vi "Autonomous Independent.vi"   [LabVIEW 2019]
doc: "This VI is called when autonomous begins, and will automatically be terminated when autonomous ends. You can carry out timed or sensor driven robot movement independently without needing to return to the caller."
uses:
  <vilib>/Rock Robotics/WPI/SafetyOutput/WPI_SafetyOutputConfigMenu.ctl
  <vilib>/Rock Robotics/WPI/Solenoid/WPI_SolenoidValue.ctl
  <vilib>/Rock Robotics/WPI/Utilities/WPI_GetSetVariantRefNum.vi
  <vilib>/Rock Robotics/Network Tables/NT Read String.vi
  <vilib>/Rock Robotics/Network Tables/NT Write Numeric Array.vi
  <vilib>/Rock Robotics/WPI/Solenoid/WPI_SolenoidSetEnum.vi
  <vilib>/Rock Robotics/WPI/RobotDrive/WPI_RobotDriveArcadeDrive_Standard(NoSaturation).vi
panel:
  # "Be sure to right-click and choose Data Operations>>Make Current Value default if you want to save the array values with the VI"
types:
  T1 = typedef "WPI_JoystickDevRef.ctl" = cluster{"Device":T2}
  T2 = typedef "WPI_JoystickDeviceEnum.ctl" = enum16{"USB 0", "USB 1", "USB 2", "USB 3", "USB 4", "USB 5"}
  T3 = typedef "WPI_SafetyOutputConfigMenu.ctl" = enum16{"Enable", "Disable"}
  T4 = typedef "WPI_SolenoidValue.ctl" = enum16{"Off", "On", "Forward", "Reverse"}
  T5 = typedef "WPI_RobotDriveDevRef.ctl" = cluster{"DevStatus":errorcluster, "Motors[]":T6[], "Square Inputs":bool, "Max Output":dbl}
  T6 = typedef "WPI_MotorControlDeviceRef.ctl" = cluster{"DeviceStatus":errorcluster, "Type":T7, "PWM":cluster{"PWM Channel":T8, "DeadBand":T9}, "CAN":cluster{"Device Number":u8, "SetOutput VI Ref":variant, "GetOutput VI Ref":variant, "Enable VI Ref":variant, "Disable VI Ref":variant, "Data":variant}, "Invert":bool, "DIO PWM":cluster{"PWM \"Enable\" Channel":T8, "DIOChannel":T10, "PWM Rate":dbl}}
  T7 = typedef "WPI_MotorControlType.ctl" = enum16{"PWM", "CAN", "DIO PWM"}
  T8 = typedef "FPGA_DIOPWMChannel.ctl" = enum8{"PWM 0", "PWM 1", "PWM 2", "PWM 3", "PWM 4", "PWM 5", "PWM 6", "PWM 7", "PWM 8", "PWM 9", "PWM MXP 0", "PWM MXP 1", "PWM MXP 2", "PWM MXP 3", "PWM MXP 4", "PWM MXP 5", "PWM MXP 6", "PWM MXP 7", "PWM MXP 8", "PWM MXP 9", "Invalid"}
  T9 = typedef "WPI_PWMDeadband.ctl" = cluster{"Name":string, "maxPositivePwm":i32, "minPositivePwm":i32, "centerPwm":i32, "maxNegativePwm":i32, "minNegativePwm":i32, "angularRange":u16}
  T10 = typedef "FPGA_DIOChannel.ctl" = enum8{"DIO 0", "DIO 1", "DIO 2", "DIO 3", "DIO 4", "DIO 5", "DIO 6", "DIO 7", "DIO 8", "DIO 9", "DIO MXP 0", "DIO MXP 1", "DIO MXP 2", "DIO MXP 3", "DIO MXP 4", "DIO MXP 5", "DIO MXP 6", "DIO MXP 7", "DIO MXP 8", "DIO MXP 9", "DIO MXP 10", "DIO MXP 11", "DIO MXP 12", "DIO MXP 13", "DIO MXP 14", "DIO MXP 15", "SPI Port CS1", "SPI Port CS2", "SPI Port CS3", "SPI Port MISO", "SPI Port MOSI", "Invalid"}
  T11 = typedef "WPI_SolenoidDevRef.ctl" = cluster{"DevStatus":errorcluster, "Pneumatics Control Module":u8, "Forward Solenoid Channel":T12, "Reverse Solenoid Channel":T12}
  T12 = typedef "WPI_SolenoidChannel.ctl" = enum8{"Solenoid 0", "Solenoid 1", "Solenoid 2", "Solenoid 3", "Solenoid 4", "Solenoid 5", "Solenoid 6", "Solenoid 7", "Invalid"}
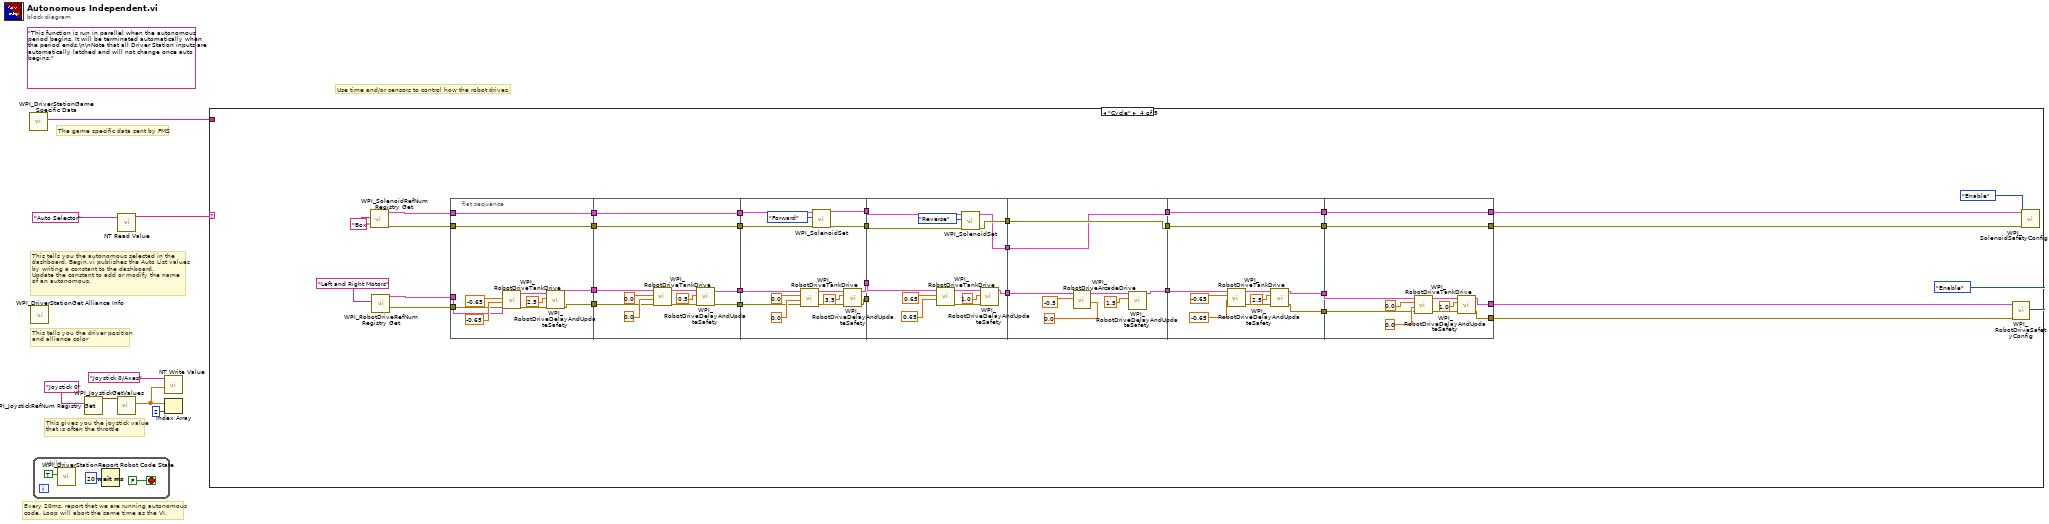
[diagram p0: block diagram]
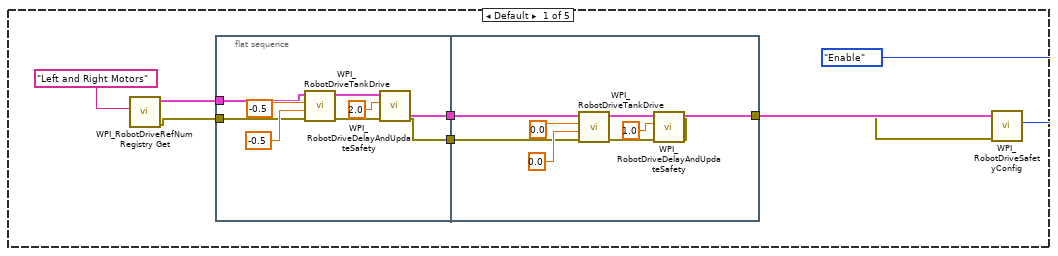
[diagram p2: hidden frame]
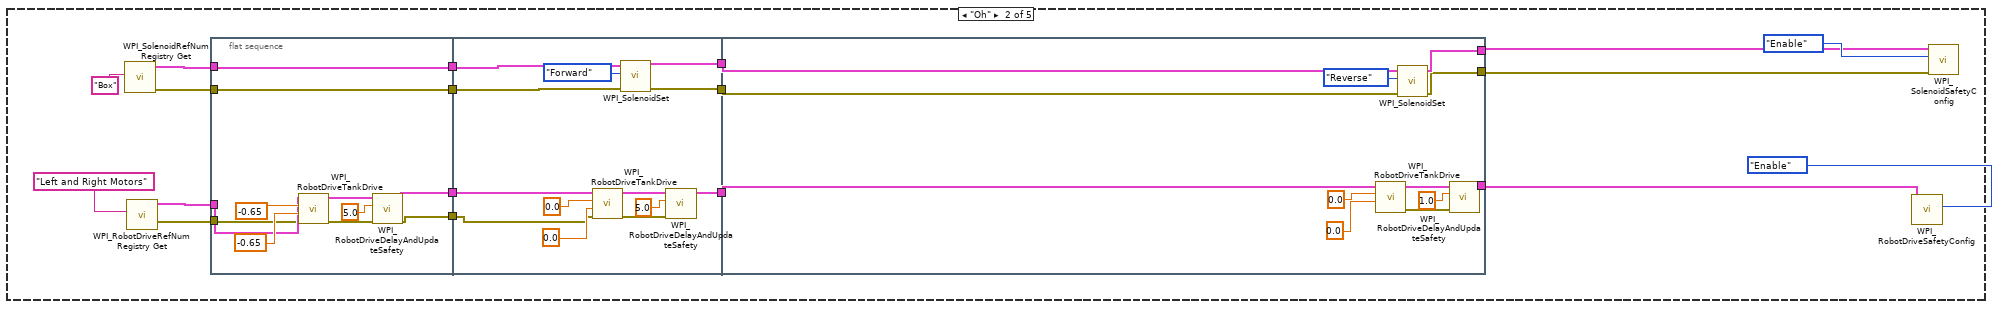
[diagram p3: hidden frame]
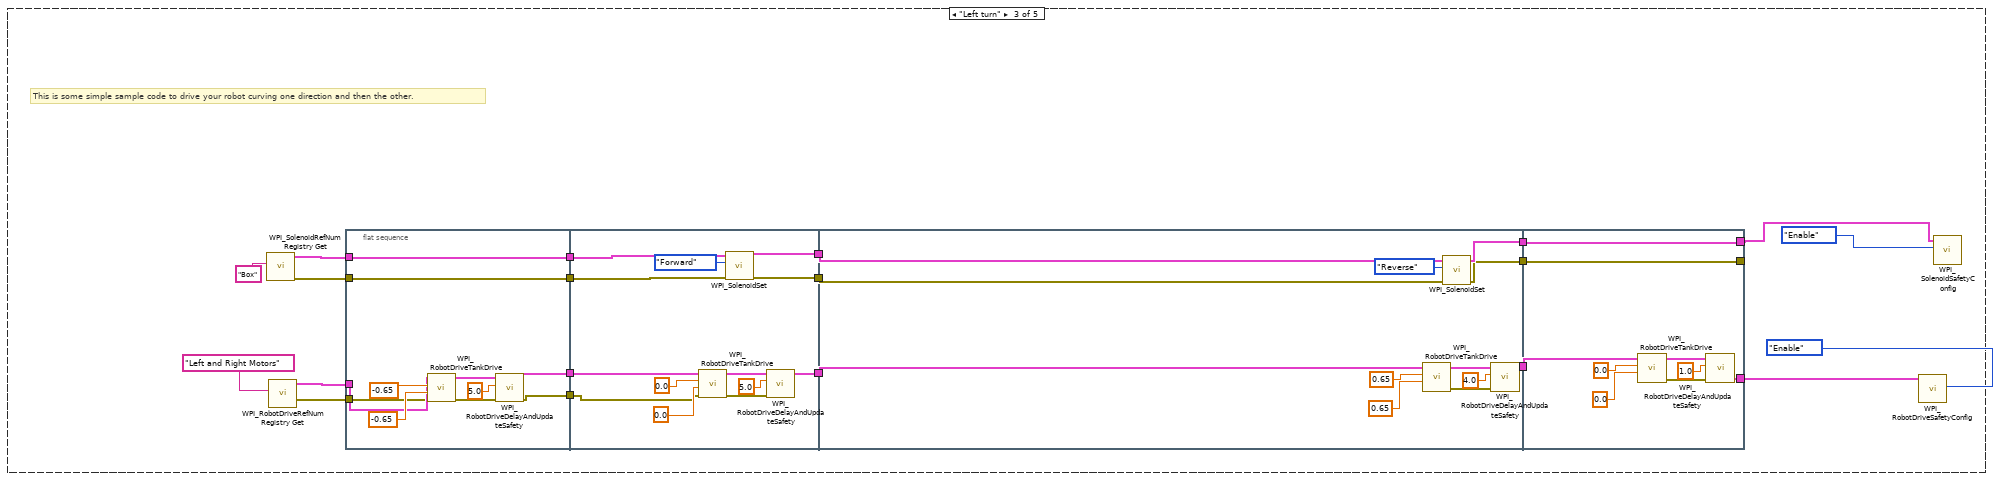
[diagram p4: hidden frame]
diagram:
  (unwired) "This function is run in parallel when the autonomous period begins. It will be terminated automatically when the period ends.\n\nNote that all Driver Station inputs are automatically latched and will not change once auto begins."
  # "The game specific data sent by FMS"
  # "This tells you the autonomous selected in the \ndashboard. Begin.vi publishes the Auto List values\nby writing a constant to the dashboard.\nUpdate the constant to add or modify the name\nof an autonomous."
  # "Every 20ms, report that we are running autonomous\ncode. Loop will abort the same time as the VI."
  # "This gives you the joystick value\nthat is often the throttle"
  # "Use time and/or sensors to control how the robot drives."
  # "This tells you the driver position\nand alliance color"
  n1 = call <vilib>:"WPI_DriverStationGame Specific Data.vi"() -> ("Game Specific Data"=w1:string)  [unwired: 11 in]
  n2 = call <vilib>:"WPI_DriverStationGet Alliance Info.vi"() -> ()  [unwired: 12 out]
  n3 = while {
    stop <- FALSE stop-if-true
    n4 = call <vilib>:"WPI_DriverStationReport Robot Code State.vi"("Autonomous"=TRUE) -> ()  [unwired: 10 in, 1 out]
    n5 = Wait (ms)(milliseconds to wait=u32 20) -> ()  [unwired: 1 out]
  }
  n6 = call <vilib>:"WPI_JoystickRefNum Registry Get.vi"("refnum name"="Joystick 0") -> ("JoystickDevRef"=w7:T1)  [unwired: 1 in, 9 out]
  n7 = call <vilib>:"WPI_JoystickGetValues.vi"("JoystickDevRef"=w7) -> ("Axes"=w3:dbl[])  [unwired: 6 in, 4 out]
  n8 = call-poly <vilib>:"NT Read Value.vi"("Name"="Auto Selector") -> ("String"=w4:string)  [unwired: 9 in, 1 out]
  n9 = call-poly <vilib>:"NT Write Value.vi"("Numeric Array"=w3, "Name"="Joystick 0/Axes") -> ()  [unwired: 9 in, 1 out]
  n10 = Index Array(array=w3, index=2) -> ()  [unwired: 1 out]
  n11 = case shown="\"Cycle\"" w4 {
    tunnel: w1 -> [_ _ _ _ _]
    frame Default {
      n12 = call <vilib>:"WPI_RobotDriveRefNum Registry Get.vi"("refnum name"="Left and Right Motors") -> ("error out"=w12:errorcluster, "RobotDriveDevRef"=w18:T5)  [unwired: 1 in, 8 out]
      n13 = flat-sequence {
        tunnel: w18 -> [w23]
        tunnel: [w22] -> w17
        tunnel: [w21] -> w13
        tunnel: w12 -> [w20]
        tunnel: w17 -> [w32]
        tunnel: [w31] -> w15
        tunnel: [w30] -> w14
        tunnel: w13 -> [w29]
        frame #0 {
          n14 = call <vilib>:"WPI_RobotDriveTankDrive.vi"("error in (no error)"=w20, "Right axis value"=-0.5 ("X axis value"), "Left axis value"=-0.5 ("X axis value"), "RobotDriveDevRef"=w23) -> ("error out"=w24:errorcluster, "RobotDriveDevRef"=w27:T5)  [unwired: 5 in, 1 out]
          n15 = call <vilib>:"WPI_RobotDriveDelayAndUpdateSafety.vi"("error in (no error)"=w24, "Delay (s)"=2.0, "RobotDriveDevRef"=w27) -> ("error out"=w21:errorcluster, "RobotDriveDevRef 2"=w22:T5)  [unwired: 7 in]
        }
        frame #1 {
          n16 = call <vilib>:"WPI_RobotDriveTankDrive.vi"("error in (no error)"=w29, "Right axis value"=0.0 ("X axis value"), "Left axis value"=0.0 ("X axis value"), "RobotDriveDevRef"=w32) -> ("error out"=w33:errorcluster, "RobotDriveDevRef"=w36:T5)  [unwired: 5 in, 1 out]
          n17 = call <vilib>:"WPI_RobotDriveDelayAndUpdateSafety.vi"("error in (no error)"=w33, "Delay (s)"=1.0, "RobotDriveDevRef"=w36) -> ("error out"=w30:errorcluster, "RobotDriveDevRef 2"=w31:T5)  [unwired: 7 in]
        }
      }
      n18 = call <vilib>:"WPI_RobotDriveSafetyConfig.vi"("error in (no error)"=w14, "mode"=WPI_SafetyOutputConfigMenu."Enable", "RobotDriveDevRef"=w15) -> ()  [unwired: 7 in, 2 out]
    }
    frame "Oh" {
      n19 = call <vilib>:"WPI_SolenoidRefNum Registry Get.vi"("refnum name"="Box") -> ("error out"=w43:errorcluster, "SolenoidDevRef"=w52:T11)  [unwired: 9 in]
      n20 = call <vilib>:"WPI_RobotDriveRefNum Registry Get.vi"("refnum name"="Left and Right Motors") -> ("error out"=w45:errorcluster, "RobotDriveDevRef"=w53:T5)  [unwired: 1 in, 8 out]
      n21 = flat-sequence {
        tunnel: w53 -> [w61]
        tunnel: w52 -> [w60]
        tunnel: [w60] -> w51
        tunnel: [w59] -> w50
        tunnel: [w58] -> w46
        tunnel: w45 -> [w57]
        tunnel: [w56] -> w44
        tunnel: w43 -> [w56]
        tunnel: [w78] -> w49
        tunnel: [w76] -> w42
        tunnel: [w69] -> w40
        tunnel: w44 -> [w77]
        tunnel: w46 -> [w67]
        tunnel: w50 -> [w70]
        tunnel: w51 -> [w79]
        tunnel: [w85] -> w41
        tunnel: [w84] -> w39
        tunnel: [w83] -> w38
        tunnel: w49 -> [w82]
        tunnel: w42 -> [w80]
        tunnel: w40 -> [w81]
        frame #0 {
          n22 = call <vilib>:"WPI_RobotDriveTankDrive.vi"("error in (no error)"=w57, "Right axis value"=-0.65 ("X axis value"), "Left axis value"=-0.65 ("X axis value"), "RobotDriveDevRef"=w61) -> ("error out"=w62:errorcluster, "RobotDriveDevRef"=w65:T5)  [unwired: 5 in, 1 out]
          n23 = call <vilib>:"WPI_RobotDriveDelayAndUpdateSafety.vi"("error in (no error)"=w62, "Delay (s)"=5.0, "RobotDriveDevRef"=w65) -> ("error out"=w58:errorcluster, "RobotDriveDevRef 2"=w59:T5)  [unwired: 7 in]
        }
        frame #1 {
          n24 = call <vilib>:"WPI_RobotDriveTankDrive.vi"("error in (no error)"=w67, "Right axis value"=0.0 ("X axis value"), "Left axis value"=0.0 ("X axis value"), "RobotDriveDevRef"=w70) -> ("error out"=w75:errorcluster, "RobotDriveDevRef"=w74:T5)  [unwired: 5 in, 1 out]
          n25 = call-poly <vilib>:"WPI_SolenoidSet.vi"("error in (no error)"=w77, "Value"=WPI_SolenoidValue."Forward", "SolenoidDevRef"=w79) -> ("error out"=w76:errorcluster, "SolenoidDevRef"=w78:T11)  [unwired: 7 in]
          n26 = call <vilib>:"WPI_RobotDriveDelayAndUpdateSafety.vi"("error in (no error)"=w75, "Delay (s)"=5.0, "RobotDriveDevRef"=w74) -> ("RobotDriveDevRef 2"=w69:T5)  [unwired: 7 in, 1 out]
        }
        frame #2 {
          n27 = call <vilib>:"WPI_RobotDriveTankDrive.vi"("Right axis value"=0.0 ("X axis value"), "Left axis value"=0.0 ("X axis value"), "RobotDriveDevRef"=w81) -> ("error out"=w90:errorcluster, "RobotDriveDevRef"=w89:T5)  [unwired: 6 in, 1 out]
          n28 = call-poly <vilib>:"WPI_SolenoidSet.vi"("error in (no error)"=w80, "Value"=WPI_SolenoidValue."Reverse", "SolenoidDevRef"=w82) -> ("error out"=w83:errorcluster, "SolenoidDevRef"=w85:T11)  [unwired: 7 in]
          n29 = call <vilib>:"WPI_RobotDriveDelayAndUpdateSafety.vi"("error in (no error)"=w90, "Delay (s)"=1.0, "RobotDriveDevRef"=w89) -> ("RobotDriveDevRef 2"=w84:T5)  [unwired: 7 in, 1 out]
        }
      }
      n30 = call <vilib>:"WPI_RobotDriveSafetyConfig.vi"("mode"=WPI_SafetyOutputConfigMenu."Enable", "RobotDriveDevRef"=w39) -> ()  [unwired: 8 in, 2 out]
      n31 = call <vilib>:"WPI_SolenoidSafetyConfig.vi"("error in (no error)"=w38, "mode"=WPI_SafetyOutputConfigMenu."Enable", "SolenoidDevRef"=w41) -> ()  [unwired: 7 in, 2 out]
    }
    frame "Left turn" {
      # "This is some simple sample code to drive your robot curving one direction and then the other."
      n32 = call <vilib>:"WPI_SolenoidRefNum Registry Get.vi"("refnum name"="Box") -> ("error out"=w97:errorcluster, "SolenoidDevRef"=w101:T11)  [unwired: 9 in]
      n33 = call <vilib>:"WPI_RobotDriveRefNum Registry Get.vi"("refnum name"="Left and Right Motors") -> ("error out"=w98:errorcluster, "RobotDriveDevRef"=w102:T5)  [unwired: 1 in, 8 out]
      n34 = flat-sequence {
        tunnel: w102 -> [w117]
        tunnel: w101 -> [w116]
        tunnel: [w116] -> w108
        tunnel: [w115] -> w109
        tunnel: [w114] -> w110
        tunnel: w98 -> [w113]
        tunnel: [w112] -> w111
        tunnel: w97 -> [w112]
        tunnel: [w134] -> w107
        tunnel: [w132] -> w106
        tunnel: [w125] -> w105
        tunnel: w111 -> [w133]
        tunnel: w110 -> [w123]
        tunnel: w109 -> [w126]
        tunnel: w108 -> [w135]
        tunnel: w107 -> [w138]
        tunnel: w106 -> [w136]
        tunnel: w105 -> [w137]
        tunnel: [w141] -> w96
        tunnel: [w140] -> w95
        tunnel: [w139] -> w94
        tunnel: [w155] -> _
        tunnel: [w156] -> w93
        tunnel: w96 -> [w156]
        tunnel: w95 -> [w149]
        tunnel: w94 -> [w155]
        tunnel: [w148] -> w92
        frame #0 {
          n35 = call <vilib>:"WPI_RobotDriveTankDrive.vi"("error in (no error)"=w113, "Right axis value"=-0.65 ("X axis value"), "Left axis value"=-0.65 ("X axis value"), "RobotDriveDevRef"=w117) -> ("error out"=w118:errorcluster, "RobotDriveDevRef"=w121:T5)  [unwired: 5 in, 1 out]
          n36 = call <vilib>:"WPI_RobotDriveDelayAndUpdateSafety.vi"("error in (no error)"=w118, "Delay (s)"=5.0, "RobotDriveDevRef"=w121) -> ("error out"=w114:errorcluster, "RobotDriveDevRef 2"=w115:T5)  [unwired: 7 in]
        }
        frame #1 {
          n37 = call <vilib>:"WPI_RobotDriveTankDrive.vi"("error in (no error)"=w123, "Right axis value"=0.0 ("X axis value"), "Left axis value"=0.0 ("X axis value"), "RobotDriveDevRef"=w126) -> ("error out"=w131:errorcluster, "RobotDriveDevRef"=w130:T5)  [unwired: 5 in, 1 out]
          n38 = call-poly <vilib>:"WPI_SolenoidSet.vi"("error in (no error)"=w133, "Value"=WPI_SolenoidValue."Forward", "SolenoidDevRef"=w135) -> ("error out"=w132:errorcluster, "SolenoidDevRef"=w134:T11)  [unwired: 7 in]
          n39 = call <vilib>:"WPI_RobotDriveDelayAndUpdateSafety.vi"("error in (no error)"=w131, "Delay (s)"=5.0, "RobotDriveDevRef"=w130) -> ("RobotDriveDevRef 2"=w125:T5)  [unwired: 7 in, 1 out]
        }
        frame #2 {
          n40 = call <vilib>:"WPI_RobotDriveTankDrive.vi"("Right axis value"=0.65 ("X axis value"), "Left axis value"=0.65 ("X axis value"), "RobotDriveDevRef"=w137) -> ("error out"=w146:errorcluster, "RobotDriveDevRef"=w145:T5)  [unwired: 6 in, 1 out]
          n41 = call-poly <vilib>:"WPI_SolenoidSet.vi"("error in (no error)"=w136, "Value"=WPI_SolenoidValue."Reverse", "SolenoidDevRef"=w138) -> ("error out"=w139:errorcluster, "SolenoidDevRef"=w141:T11)  [unwired: 7 in]
          n42 = call <vilib>:"WPI_RobotDriveDelayAndUpdateSafety.vi"("error in (no error)"=w146, "Delay (s)"=4.0, "RobotDriveDevRef"=w145) -> ("RobotDriveDevRef 2"=w140:T5)  [unwired: 7 in, 1 out]
        }
        frame #3 {
          n43 = call <vilib>:"WPI_RobotDriveTankDrive.vi"("Right axis value"=0.0 ("X axis value"), "Left axis value"=0.0 ("X axis value"), "RobotDriveDevRef"=w149) -> ("error out"=w154:errorcluster, "RobotDriveDevRef"=w153:T5)  [unwired: 6 in, 1 out]
          n44 = call <vilib>:"WPI_RobotDriveDelayAndUpdateSafety.vi"("error in (no error)"=w154, "Delay (s)"=1.0, "RobotDriveDevRef"=w153) -> ("RobotDriveDevRef 2"=w148:T5)  [unwired: 7 in, 1 out]
        }
      }
      n45 = call <vilib>:"WPI_RobotDriveSafetyConfig.vi"("mode"=WPI_SafetyOutputConfigMenu."Enable", "RobotDriveDevRef"=w92) -> ()  [unwired: 8 in, 2 out]
      n46 = call <vilib>:"WPI_SolenoidSafetyConfig.vi"("mode"=WPI_SafetyOutputConfigMenu."Enable", "SolenoidDevRef"=w93) -> ()  [unwired: 8 in, 2 out]
    }
    frame "Cycle" {
      n47 = call <vilib>:"WPI_SolenoidRefNum Registry Get.vi"("refnum name"="Box") -> ("error out"=w175:errorcluster, "SolenoidDevRef"=w183:T11)  [unwired: 9 in]
      n48 = call <vilib>:"WPI_RobotDriveRefNum Registry Get.vi"("refnum name"="Left and Right Motors") -> ("error out"=w178:errorcluster, "RobotDriveDevRef"=w184:T5)  [unwired: 1 in, 8 out]
      n49 = flat-sequence {
        tunnel: w184 -> [w196]
        tunnel: w183 -> [w195]
        tunnel: [w195] -> w190
        tunnel: [w194] -> w189
        tunnel: [w193] -> w179
        tunnel: w178 -> [w192]
        tunnel: [w191] -> w176
        tunnel: w175 -> [w191]
        tunnel: w190 -> [w206]
        tunnel: w189 -> [w207]
        tunnel: [w206] -> w188
        tunnel: [w205] -> w187
        tunnel: [w204] -> w180
        tunnel: w179 -> [w203]
        tunnel: [w202] -> w177
        tunnel: w176 -> [w202]
        tunnel: w188 -> [w219]
        tunnel: w187 -> [w221]
        tunnel: [w218] -> w161
        tunnel: [w217] -> w162
        tunnel: [w216] -> w163
        tunnel: w180 -> [w215]
        tunnel: w177 -> [w214]
        tunnel: [w213] -> w164
        tunnel: w164 -> [w234]
        tunnel: w163 -> [_]
        tunnel: w162 -> [w227]
        tunnel: w161 -> [w235]
        tunnel: [w237] -> w160
        tunnel: [w236] -> w159
        tunnel: [w228] -> w158
        tunnel: [w242] -> w174
        tunnel: [w240] -> w170
        tunnel: [w241] -> w167
        tunnel: w160 -> [w241]
        tunnel: w159 -> [w240]
        tunnel: w158 -> [w239]
        tunnel: w174 -> [w252]
        tunnel: [w250] -> w173
        tunnel: [w249] -> w171
        tunnel: w170 -> [w249]
        tunnel: [w248] -> w168
        tunnel: w167 -> [w248]
        tunnel: [w247] -> w157
        tunnel: [w262] -> w172
        tunnel: [w261] -> w169
        tunnel: [w260] -> w166
        tunnel: [w259] -> w165
        tunnel: w173 -> [w258]
        tunnel: w171 -> [w262]
        tunnel: w168 -> [w261]
        tunnel: w157 -> [w257]
        frame #0 {
          n50 = call <vilib>:"WPI_RobotDriveTankDrive.vi"("error in (no error)"=w192, "Right axis value"=-0.65 ("X axis value"), "Left axis value"=-0.65 ("X axis value"), "RobotDriveDevRef"=w196) -> ("error out"=w197:errorcluster, "RobotDriveDevRef"=w200:T5)  [unwired: 5 in, 1 out]
          n51 = call <vilib>:"WPI_RobotDriveDelayAndUpdateSafety.vi"("error in (no error)"=w197, "Delay (s)"=2.5, "RobotDriveDevRef"=w200) -> ("error out"=w193:errorcluster, "RobotDriveDevRef 2"=w194:T5)  [unwired: 7 in]
        }
        frame #1 {
          n52 = call <vilib>:"WPI_RobotDriveTankDrive.vi"("error in (no error)"=w203, "Right axis value"=0.0 ("X axis value"), "Left axis value"=0.0 ("X axis value"), "RobotDriveDevRef"=w207) -> ("error out"=w208:errorcluster, "RobotDriveDevRef"=w211:T5)  [unwired: 5 in, 1 out]
          n53 = call <vilib>:"WPI_RobotDriveDelayAndUpdateSafety.vi"("error in (no error)"=w208, "Delay (s)"=0.5, "RobotDriveDevRef"=w211) -> ("error out"=w204:errorcluster, "RobotDriveDevRef 2"=w205:T5)  [unwired: 7 in]
        }
        frame #2 {
          n54 = call <vilib>:"WPI_RobotDriveTankDrive.vi"("error in (no error)"=w215, "Right axis value"=0.0 ("X axis value"), "Left axis value"=0.0 ("X axis value"), "RobotDriveDevRef"=w221) -> ("error out"=w222:errorcluster, "RobotDriveDevRef"=w225:T5)  [unwired: 5 in, 1 out]
          n55 = call-poly <vilib>:"WPI_SolenoidSet.vi"("error in (no error)"=w214, "Value"=WPI_SolenoidValue."Forward", "SolenoidDevRef"=w219) -> ("error out"=w213:errorcluster, "SolenoidDevRef"=w218:T11)  [unwired: 7 in]
          n56 = call <vilib>:"WPI_RobotDriveDelayAndUpdateSafety.vi"("error in (no error)"=w222, "Delay (s)"=3.5, "RobotDriveDevRef"=w225) -> ("error out"=w216:errorcluster, "RobotDriveDevRef 2"=w217:T5)  [unwired: 7 in]
        }
        frame #3 {
          n57 = call <vilib>:"WPI_RobotDriveTankDrive.vi"("Right axis value"=0.65 ("X axis value"), "Left axis value"=0.65 ("X axis value"), "RobotDriveDevRef"=w227) -> ("error out"=w229:errorcluster, "RobotDriveDevRef"=w232:T5)  [unwired: 6 in, 1 out]
          n58 = call-poly <vilib>:"WPI_SolenoidSet.vi"("error in (no error)"=w234, "Value"=WPI_SolenoidValue."Reverse", "SolenoidDevRef"=w235) -> ("error out"=w237:errorcluster, "SolenoidDevRef"=w236:T11)  [unwired: 7 in]
          n59 = call <vilib>:"WPI_RobotDriveDelayAndUpdateSafety.vi"("error in (no error)"=w229, "Delay (s)"=1.0, "RobotDriveDevRef"=w232) -> ("RobotDriveDevRef 2"=w228:T5)  [unwired: 7 in, 1 out]
        }
        frame #4 {
          n60 = call-poly <vilib>:"WPI_RobotDriveArcadeDrive.vi"("Y axis value"=0.0 ("X axis value"), "X axis value"=-0.5, "RobotDriveDevRef"=w239) -> ("RobotDriveDevRef"=w246:T5)  [unwired: 6 in, 2 out]
          n61 = call <vilib>:"WPI_RobotDriveDelayAndUpdateSafety.vi"("Delay (s)"=1.5, "RobotDriveDevRef"=w246) -> ("RobotDriveDevRef 2"=w242:T5)  [unwired: 8 in, 1 out]
        }
        frame #5 {
          n62 = call <vilib>:"WPI_RobotDriveTankDrive.vi"("Right axis value"=-0.65 ("X axis value"), "Left axis value"=-0.65 ("X axis value"), "RobotDriveDevRef"=w252) -> ("error out"=w253:errorcluster, "RobotDriveDevRef"=w255:T5)  [unwired: 6 in, 1 out]
          n63 = call <vilib>:"WPI_RobotDriveDelayAndUpdateSafety.vi"("error in (no error)"=w253, "Delay (s)"=2.5, "RobotDriveDevRef"=w255) -> ("error out"=w247:errorcluster, "RobotDriveDevRef 2"=w250:T5)  [unwired: 7 in]
        }
        frame #6 {
          n64 = call <vilib>:"WPI_RobotDriveTankDrive.vi"("error in (no error)"=w257, "Right axis value"=0.0 ("X axis value"), "Left axis value"=0.0 ("X axis value"), "RobotDriveDevRef"=w258) -> ("error out"=w267:errorcluster, "RobotDriveDevRef"=w266:T5)  [unwired: 5 in, 1 out]
          n65 = call <vilib>:"WPI_RobotDriveDelayAndUpdateSafety.vi"("error in (no error)"=w267, "Delay (s)"=1.0, "RobotDriveDevRef"=w266) -> ("error out"=w259:errorcluster, "RobotDriveDevRef 2"=w260:T5)  [unwired: 7 in]
        }
      }
      n66 = call <vilib>:"WPI_RobotDriveSafetyConfig.vi"("error in (no error)"=w165, "mode"=WPI_SafetyOutputConfigMenu."Enable", "RobotDriveDevRef"=w166) -> ()  [unwired: 7 in, 2 out]
      n67 = call <vilib>:"WPI_SolenoidSafetyConfig.vi"("error in (no error)"=w169, "mode"=WPI_SafetyOutputConfigMenu."Enable", "SolenoidDevRef"=w172) -> ()  [unwired: 7 in, 2 out]
    }
    frame "Your Turn" {
    }
  }
